vi "drive.vi"(8 "distance":dbl=100.0, 9 "Y":dbl=-1.0, 10 "X":dbl, 11 "RobotDriveDevRef":T1={"DevStatus"={"status"=FALSE, "code"=0, "source"=""}, "Motors[]"=[], "Square Inputs"=FALSE, "Max Output"=1.0}) -> (3 "RobotDriveDevRef dup.":T1={"DevStatus"={"status"=FALSE, "code"=0, "source"=""}, "Motors[]"=[], "Square Inputs"=FALSE, "Max Output"=1.0})   [LabVIEW 2016]
uses:
  <vilib>/Rock Robotics/WPI/RobotDrive/WPI_RobotDriveDevRef.ctl
  <vilib>/Rock Robotics/WPI/MotorControl/WPI_MotorControlDeviceRef.ctl
  <vilib>/Rock Robotics/WPI/MotorControl/WPI_MotorControlType.ctl
  <vilib>/Rock Robotics/SystemInterfaces/DIO/FPGA_DIOPWMChannel.ctl
  <vilib>/Rock Robotics/WPI/PWM/WPI_PWMDeadband.ctl
  <vilib>/Rock Robotics/Network Tables/NT Write Number.vi
  <vilib>/Rock Robotics/WPI/RobotDrive/WPI_RobotDriveArcadeDrive_Standard(NoSaturation).vi
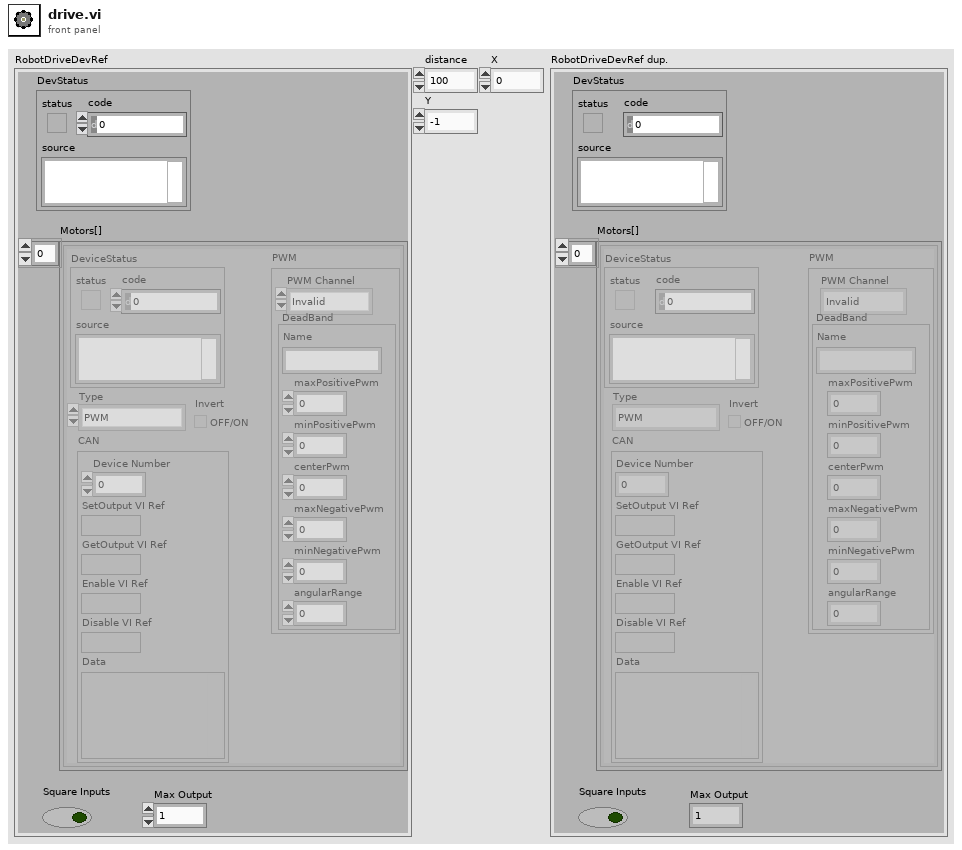
[diagram p1: front panel]
types:
  T1 = typedef "WPI_RobotDriveDevRef.ctl" = cluster{"DevStatus":errorcluster, "Motors[]":T2[], "Square Inputs":bool, "Max Output":dbl}
  T2 = typedef "WPI_MotorControlDeviceRef.ctl" = cluster{"DeviceStatus":errorcluster, "Type":T3, "PWM":cluster{"PWM Channel":T4, "DeadBand":T5}, "CAN":cluster{"Device Number":u8, "SetOutput VI Ref":variant, "GetOutput VI Ref":variant, "Enable VI Ref":variant, "Disable VI Ref":variant, "Data":variant}, "Invert":bool}
  T3 = typedef "WPI_MotorControlType.ctl" = enum16{"PWM", "CAN"}
  T4 = typedef "FPGA_DIOPWMChannel.ctl" = enum8{"PWM 0", "PWM 1", "PWM 2", "PWM 3", "PWM 4", "PWM 5", "PWM 6", "PWM 7", "PWM 8", "PWM 9", "PWM MXP 0", "PWM MXP 1", "PWM MXP 2", "PWM MXP 3", "PWM MXP 4", "PWM MXP 5", "PWM MXP 6", "PWM MXP 7", "PWM MXP 8", "PWM MXP 9", "Invalid"}
  T5 = typedef "WPI_PWMDeadband.ctl" = cluster{"Name":string, "maxPositivePwm":i32, "minPositivePwm":i32, "centerPwm":i32, "maxNegativePwm":i32, "minNegativePwm":i32, "angularRange":u16}
  T6 = typedef "WPI_CANJaguar_Status.ctl" = cluster{"Output Percent VBus":dbl, "Output Voltage":dbl, "Bus Voltage":dbl, "Current":dbl, "Temperature":dbl, "Position":dbl, "Speed":dbl, "Limits":cluster{"Forward Limit":bool, "Reverse Limit":bool, "Forward Soft Limit":bool, "Reverse Soft Limit":bool, "Sticky Forward Limit":bool, "Sticky Reverse Limit":bool, "Sticky Forward Soft Limit":bool, "Sticky Reverse Soft Limit":bool}, "Faults":cluster{"Current Fault":bool, "Temperature Fault":bool, "Bus Voltage Fault":bool, "Gate Driver Fault":bool, "Comm Fault":bool}, "Fault Counters":cluster{"Current Faults":u8, "Temperature Faults":u8, "Bus Voltage Faults":u8, "Gate Driver Faults":u8, "Comm Faults":u8, "CAN Status":u8, "CAN RX Errors":u8, "CAN TX Errors":u8}, "Power Cycle":bool}
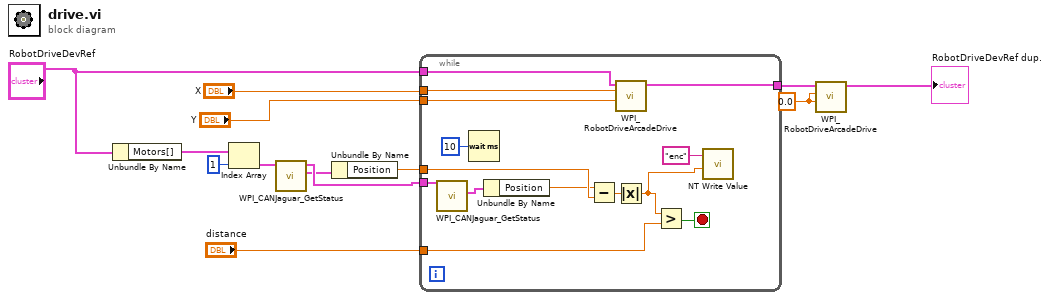
[diagram p0: block diagram]
diagram:
  w5 = 0.0 ("Y axis value")
  n1 = Unbundle By Name("RobotDriveDevRef") -> ("Motors[]"=w12:T2[])
  n2 = Index Array(array=w12, index=1) -> (element=w4:T2)
  n3 = call <vilib>:"WPI_CANJaguar_GetStatus.vi"("CAN Jaguar Ref"=w4) -> ("Status"=w2:T6, "CAN Jaguar Ref"=w3:T2)  [unwired: 8 in, 1 out]
  n4 = Unbundle By Name(w2) -> ("Position"=w1:dbl)
  n5 = while {
    tunnel: [w27] -> w8
    tunnel: "RobotDriveDevRef" -> [w25]
    tunnel: w3 -> [w16]
    tunnel: "X" -> [w24]
    tunnel: "Y" -> [w23]
    tunnel: "distance" -> [w22]
    tunnel: w1 -> [w17]
    stop <- w26 stop-if-true
    n6 = call <vilib>:"WPI_CANJaguar_GetStatus.vi"("CAN Jaguar Ref"=w16) -> ("Status"=w15:T6)  [unwired: 8 in, 2 out]
    n7 = Wait (ms)(milliseconds to wait=u32 10) -> ()  [unwired: 1 out]
    n8 = Unbundle By Name(w15) -> ("Position"=w14:dbl)
    n9 = Subtract(x=w14, y=w17) -> (x-y=w18:dbl)
    n10 = call-poly <vilib>:"WPI_RobotDriveArcadeDrive.vi"("Y axis value"=w23, "X axis value"=w24, "RobotDriveDevRef"=w25) -> ("RobotDriveDevRef"=w27:T1)  [unwired: 6 in, 2 out]
    n11 = Absolute Value(x=w18) -> (abs(x)=w21:dbl)
    n12 = Greater?(x=w21, y=w22) -> (0:w26:bool)
    n13 = call-poly <vilib>:"NT Write Value.vi"("Numeric"=w21, "Name"="enc") -> ()  [unwired: 9 in, 1 out]
  }
  n14 = call-poly <vilib>:"WPI_RobotDriveArcadeDrive.vi"("Y axis value"=w5, "X axis value"=w5, "RobotDriveDevRef"=w8) -> ("RobotDriveDevRef"=→"RobotDriveDevRef dup.":T1)  [unwired: 6 in, 2 out]
